vi "Initialize Shared Library.vi"(6 "Unload":bool, 8 "Error In":errorcluster, 11 "libssh2lv Shared Library In":path) -> (0 "Error Out":errorcluster, 2 "Return Code":i32, 3 "libssh2lv Shared Library Out":path)   [LabVIEW 2018, in "Toolkit.lvlib" / "SSH.lvclass"]
uses:
  SSH.lvclass
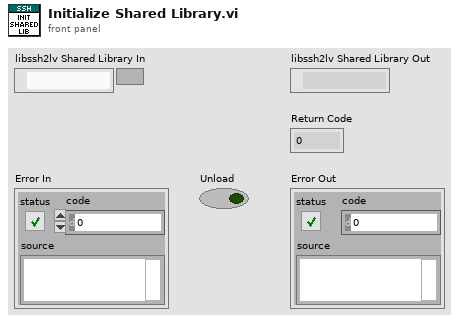
[diagram p1: front panel]
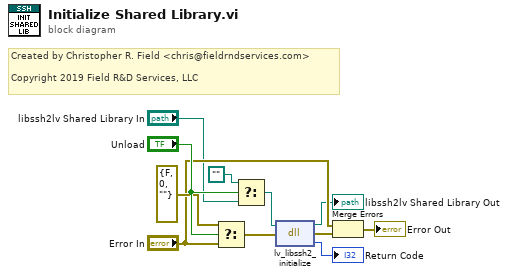
[diagram p0: block diagram]
diagram:
  # "Created by Christopher R. Field <chris@fieldrndservices.com>\n\nCopyright 2019 Field R&D Services, LLC"
  n1 = Select(t=errorcluster {"status"=FALSE, "code"=0, "source"=""} ("error out"), s="Unload", f="Error In") -> (s? t:f=w6:errorcluster)
  n2 = Select(t=path "", s="Unload", f="libssh2lv Shared Library In") -> (s? t:f=w1:path)
  n3 = dll-call lib="D:/Users/cfield/Code/Field R&D Services/SSH/LV-LIBSSH2/LabVIEW/trunk/src/Toolkit/Support/lv-libssh2.*" fn="lv_libssh2_initialize"(path in=w1, error in=w6) -> (path out=→"libssh2lv Shared Library Out":path, error out=w5:errorcluster, "return type"=→"Return Code":i32)  [unwired: 1 in]
  n4 = Merge Errors("Error In", w5) -> (→"Error Out":errorcluster)
